vi "Set System References.vi"(8 "error in (no error)":errorcluster) -> (0 "error out":errorcluster, 3 "System Resources":T1)   [LabVIEW 2020]
doc: "This VI gets the system session and system reference and puts it on the appropriate notifier."
uses:
  <vilib>/nisyscfg/nisyscfg.lvlib
  <resource>/objmgr/nisysapi.rc
  Type Definitions/System Resources.ctl
  <vilib>/rvi/interface/nirviOpenFPGA/nirviOpenFPGA.xnode
  <vilib>/rvi/interface/nirviMethod/nirviMethod.xnode
  <vilib>/FPGAPlugInAG/Dynamic/niLvFpga_Reset_Dynamic.vi
  <vilib>/FPGAPlugInAG/Dynamic/niLvFpga_Run_Dynamic.vi
  Builds/FPGA Bitfiles/Exec_FPGA.lvbitx
  <vilib>/FPGAPlugInAG/cRIO-9038/niLvFpga_Open_cRIO-9038.vi
  <vilib>/rvi/interface/common/dynamic/niFpgaDynamicAddResources.vi
  Type Definitions/Payload Class.ctl
  Type Definitions/Enum - Parameters.ctl
  <vilib>/rvi/interface/nirviReadWriteControl/nirviReadWriteControl.xnode
  NiFpgaLv.dll
  <vilib>/Utility/error.llb/Error Cluster From Error Code.vi
  <vilib>/rvi/interface/Simulation/niFpgaSimulationCallBeginRW.vi
  <vilib>/rvi/errors/niLvFpgaAdjustHostInterfaceError.vi
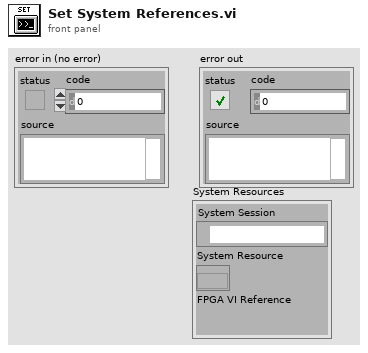
[diagram p1: front panel]
types:
  T1 = typedef "System Resources.ctl" = cluster{"System Session":refnum<k21>, "System Resource":refnum<k20>, "FPGA VI Reference":refnum<k20>}
  T2 = typedef "Enum - Parameters.ctl" = enum16{"Device Parameters"}
  T3 = typedef "Payload Class.ctl" = enum16{"System State", "Parameters", "Metadata", "Software Monitor", "Data", "Commands"}
  T4 = typedef "Device Parameters.ctl" = cluster{"Device":T5}
  T5 = typedef "Device.ctl" = enum32{"None", "Exec", "Aux1", "Aux2", "Aux3"}
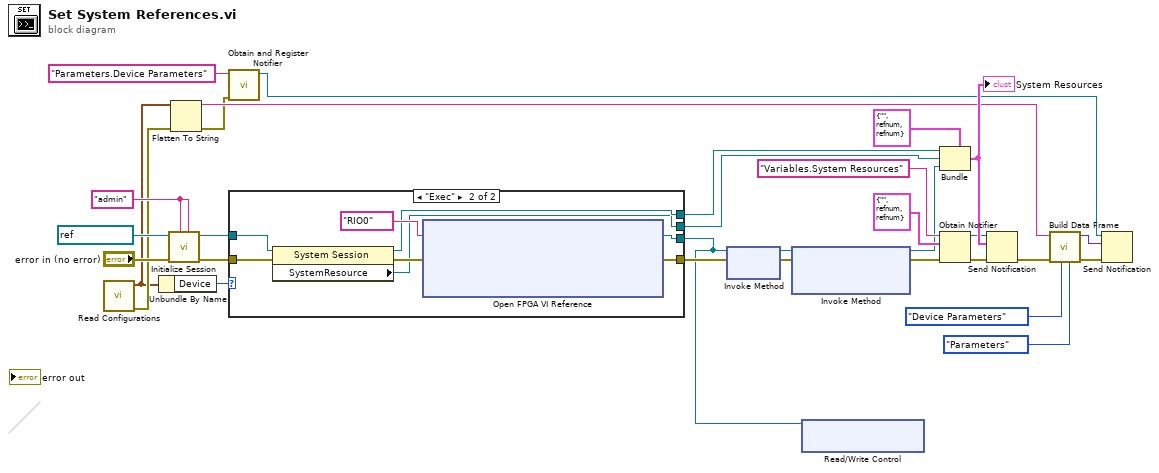
[diagram p0: block diagram]
diagram:
  w22 = "admin" ("User Name")
  n1 = call "Read Configurations.vi"() -> ("error out"=w7:errorcluster, "Device Parameters"=w4:T4)  [unwired: 10 in]
  n2 = Unbundle By Name(w4) -> ("Device"=w3:T5)
  n3 = call <vilib>:"Initialize Session.vi"("Password"=w22, "User Name"=w22, "error in (no error)"="error in (no error)", "Target (localhost)"=refnum<k21> "localhost") -> ("error out"=w24:errorcluster, "Session out"=w23:refnum<k21>)  [unwired: 6 in]
  n4 = Flatten To String(anything=w4, error in (no error)=w7) -> (data string=w9:string, error out=w5:errorcluster)  [unwired: 2 in, 1 out]
  n5 = call "Obtain and Register Notifier.vi"("error in (no error)"=w5, "name (unnamed)"="Parameters.Device Parameters") -> ("notifier out"=w12:refnum<notifier>)  [unwired: 7 in, 2 out]
  n6 = case shown="\"Exec\"" w3 {
    tunnel: w24 -> [_ w39]
    tunnel: w23 -> [_ w38]
    tunnel: [_ w35] -> w18
    tunnel: [_ w34] -> w1
    tunnel: [_ w33] -> w15
    tunnel: [_ w32] -> w14
    frame "None", Default {
    }
    frame "Exec" {
      n7 = property class="System Session"(reference=w38, error in=w39) -> (reference out=w33:refnum<k21>, error out=w37:errorcluster, "SystemResource"=w32:refnum<k20>)
      n8 = xnode "Open FPGA VI Reference"("error in"=w37, "resource name"=tag "RIO0") -> ("FPGA VI Reference Out"=w34:refnum<k20>, "error out"=w35:errorcluster)
    }
  }
  n9 = xnode "Invoke Method"("FPGA VI Reference In"=w1, "error in"=w18) -> ("FPGA VI Reference Out"=w16:refnum<k20>, "error out"=w17:errorcluster)
  n10 = xnode "Invoke Method"("FPGA VI Reference In"=w16, "error in"=w17) -> ("FPGA VI Reference Out"=w20:refnum<k20>, "error out"=w21:errorcluster)  [unwired: 1 in]
  n11 = xnode "Read/Write Control"("FPGA VI Reference In"=w1) -> ()  [unwired: 1 in, 3 out]
  n12 = Bundle(cluster=T1 {"System Session"="", "System Resource"=refnum, "FPGA VI Reference"=refnum} ("System References"), "System Session"=w15, "System Resource"=w14, "FPGA VI Reference"=w20) -> (w29:T1)
  "System Resources" <- w29
  n13 = Obtain Notifier(name (unnamed)="Variables.System Resources", notification data type=T1 {"System Session"="", "System Resource"=refnum, "FPGA VI Reference"=refnum} ("cluster"), error in (no error)=w21) -> (notifier out=w28:refnum<notifier>, error out=w31:errorcluster)  [unwired: 1 in, 1 out]
  n14 = Send Notification(notification=w29, notifier=w28, error in (no error)=w31) -> (error out=w2:errorcluster)  [unwired: 1 out]
  n15 = call "Build Data Frame.vi"("Payload Class (Data)"=Payload_Class."Parameters", "Payload ID (0)"=Enum_-_Parameters."Device Parameters" ("Parameters"), "error in (no error)"=w2, "Payload (Empty String)"=w9) -> ("error out"=w6:errorcluster, "Frame"=w8:variant)  [unwired: 6 in]
  n16 = Send Notification(notification=w8, notifier=w12, error in (no error)=w6) -> ()  [unwired: 2 out]
